vi "Dashboard Main.vi"() -> ()   [LabVIEW 2019]
uses:
  <vilib>/Utility/miscctls.llb/LVRowAndColumnTypeDef.ctl
  <vilib>/event_ctls.llb/eventvkey.ctl
  <vilib>/Rock Robotics/Network Tables/NT Read Numeric Array.vi
  <vilib>/Rock Robotics/Network Tables/NT Write Numeric Array.vi
  <vilib>/Rock Robotics/Network Tables/NT Read Boolean.vi
  <vilib>/Rock Robotics/WPI/Dashboard/WPI_DashboardLogging Global.vi
panel:
  in  "Camera Settings Right":T1={"Frame Rate"=30, "Compression"=30, "Size"=1, "DB Camera Config"=FALSE} {"Frame Rate" scale=1.0..30.0; "Compression" scale=100.0..-1.0; "Size" items=["640x480", "320x240", "160x120"]}
  in  "Camera Name Right":string(combo)="No Camera Selection"
  out "Camera Perf":string
  in  "Camera Settings":T1={"Frame Rate"=30, "Compression"=30, "Size"=1, "DB Camera Config"=FALSE} {"Frame Rate" scale=1.0..30.0; "Compression" scale=100.0..-1.0; "Size" items=["640x480", "320x240", "160x120"]}
  in  "TCP":refnum<k5>
  in  "Rec Mode":enum32{"Stop", "Record", "Playback"}(radio)
  out "Image Message":string="Timeout in Camera Communications"
  in  "Dashboard Tab":T2(tab)
  in  "Position":enum16{"", "1", "2", "3"}(ring)
  in  "Auto Route":string(combo)
  out "VisionAligned":bool
  out "NT Connection":bool
  out "Mode":T3(ring)=enum."Auto Disabled"
  out "Right Camera Perf":cluster{"Bandwidth (Mbps)":dbl, "FPS":dbl}
  in  "Write Swerve Offsets":bool
  out "Camera Image Right":T4(plugin-control)
  in  "DB/String 9":string
  in  "DB/String 8":string
  in  "DB/String 7":string
  in  "DB/String 6":string
  in  "DB/String 5":string
  in  "DB/String 4":string
  in  "DB/String 3":string
  in  "DB/String 2":string
  in  "DB/String 1":string
  in  "DB/String 0":string
  in  "DB/Slider 0":dbl(slide) scale=0.0..5.0
  in  "DB/Slider 1":dbl(slide) scale=0.0..5.0
  in  "DB/Slider 2":dbl(slide) scale=0.0..5.0
  in  "DB/Slider 3":dbl(slide) scale=0.0..5.0
  out "DB/LED 3":bool
  out "DB/LED 2":bool
  out "DB/LED 1":bool
  out "DB/LED 0":bool
  in  "DB/Button 3":bool
  in  "DB/Button 2":bool
  in  "DB/Button 1":bool
  in  "DB/Button 0":bool caption="New Name"
  in  "Test Slider":dbl(slide) scale=0.0..100.0 scale format="%#_3g"
  in  "On/Off":bool caption="Solenoid"
  in  "Test Name":u16(ring) items=["Select the test to run..."]
  in  "Test Tree":string(tree)
  in  "Motor":cluster{"Value":dbl, "Enable":bool} {"Value" scale=-1.0..1.0 scale format="%#_3g"}
  out "Progress":T5 {"Test Progress" scale=0.0..100.0}
  in  "Rev/Fwd":cluster{"Forward":bool, "Reverse":bool}
  in  "Test Ring":u16(ring) items=["Monochrome", "Color"]
  out "Cmd Status":string
  in  "Execute Command":bool
  in  "Command Params":string[][](table)
  in  "Command Selection":i32(listbox)
  in  "CheckList":i32(listbox)
  out "Tree":string(tree)
  out "Camera Image":T4(plugin-control)
  out "Background":bool
  in  "Camera Name":string(combo)="No Camera Selection"
  # "HW"
  # "HW"
  # "General"
  # "Autonomous"
  # "This tab is a great place for autonomous settings and robot-specific values.\nPlace controls and indicators inside this tab and match name to\nDashboard Variables on robot. You can also delete this comment."
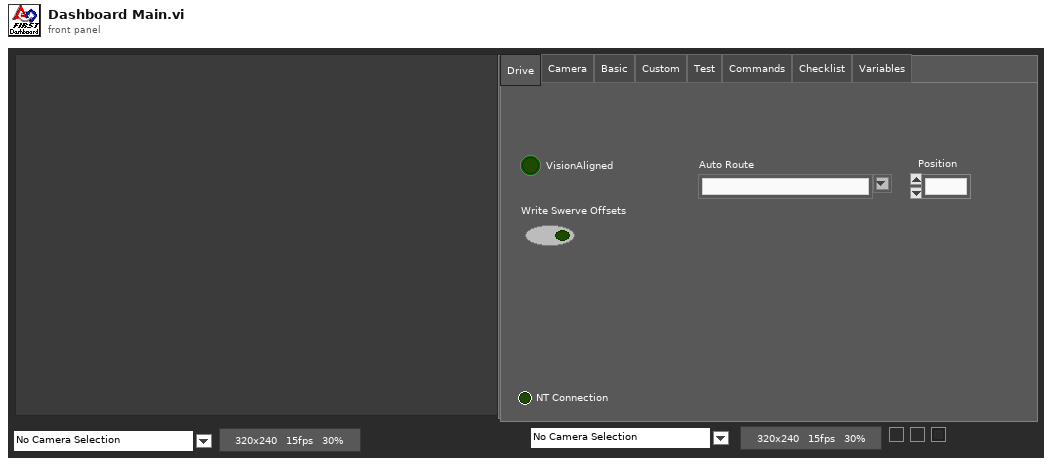
[diagram p1: front panel]
types:
  T1 = cluster{"Frame Rate":i32, "Compression":i32, "Size":u16, "DB Camera Config":bool}
  T2 = enum32{"Drive", "Camera", "Basic", "Custom", "Test", "Commands", "Checklist", "Variables"}
  T3 = enum8{"Tele-Op Disabled", "Tele-Op Enabled", "Auto Disabled", "Auto Enabled", "Test Disabled", "Test Enabled", "Disconnected", "No Code", "E-Stop"}
  T4 = typedef "IMAQ Image.ctl" = refnum<image>
  T5 = cluster{"Test Progress":u8, "Test Progress Text":string}
  T6 = cluster{"Save Path":path, "Interval (s)":dbl, "Keep":i32}
  T7 = typedef "Image Type" = u32
  T8 = cluster{"IDs":cluster{"RPC field ID":u16, "Unique ID":u16}, "String":string}
  T9 = cluster{"Camera Image":refnum<vi>, "Dashboard Tab":refnum<vi>, "Background":refnum<vi>, "Rec Mode":refnum<vi>, "Test Slider":refnum<vi>, "On/Off ":refnum<vi>, "Test Ring":refnum<vi>, "Rev/Fwd":refnum<vi>, "Test Name":refnum<vi>, "Motor":refnum<vi>, "Progress":refnum<vi>, "CheckList":refnum<vi>, "Tree":refnum<vi>, "Test Tree":refnum<vi>, "Command Params":refnum<vi>, "Command Selection":refnum<vi>, "Execute Command":refnum<vi>, "Cmd Status":refnum<vi>, "Camera Settings":refnum<vi>, "Camera Name":refnum<vi>, "Camera Perf":refnum<vi>, "Camera Settings Right":refnum<vi>, "Camera Name Right":refnum<vi>, "Camera Image Right":refnum<vi>}
  T10 = cluster{"Global Rectangle":i32[], "Contours":cluster{"Contour Type":u32, "ROI Type":u32, "Points":i32[]}[]}
  T11 = cluster{"Camera Name":string, string, "Saved DB Images Info":cluster{"Save Path":path, "Interval (s)":dbl, "Keep":i32}}
  T12 = cluster{"Camera Name Right":string, string, "Saved DB Images Info":cluster{"Save Path":path, "Interval (s)":dbl, "Keep":i32}}
  T13 = cluster{"Operation":enum16{"Update", "Clear"}, "Color Box":u32}[]
  T14 = typedef "eventvkey.ctl" = enum16{"ASCII", "Enter", "Return", "Shift", "Ctrl", "Alt", "Cmd", "Opt", "Caps", "NumLock", "Clear", "Break", "Up", "Down", "Left", "Right", "Insert", "Delete", "Home", "End", "PageUp", "PageDown", "Escape", "Help", "Pause", "ScrollLock", "F1", "F2", "F3", "F4", "F5", "F6", "F7", "F8", "F9", "F10", "F11", "F12", "F13", "F14", "F15", "F16", "F17", "F18", "F19", "F20", "F21", "F22", "F23", "F24", "Play", "VolumeUp", "VolumeDown", "Mute", "Two Byte Char"}
  T15 = cluster{"Image Size":bool, "Image Type":bool, "Pixel Value":bool, "ROI Information":bool, "Zoom Factor":bool}
  T16 = cluster{"Operation":enum16{"Update", "Clear"}, "Color Box":u32}
  T17 = typedef "LVRowAndColumnTypeDef.ctl" = cluster{"Row":i32, "Column":i32}
  T18 = cluster{"Shift":bool, "Ctrl":bool, "Alt":bool, "Cmd":bool, "Opt":bool}
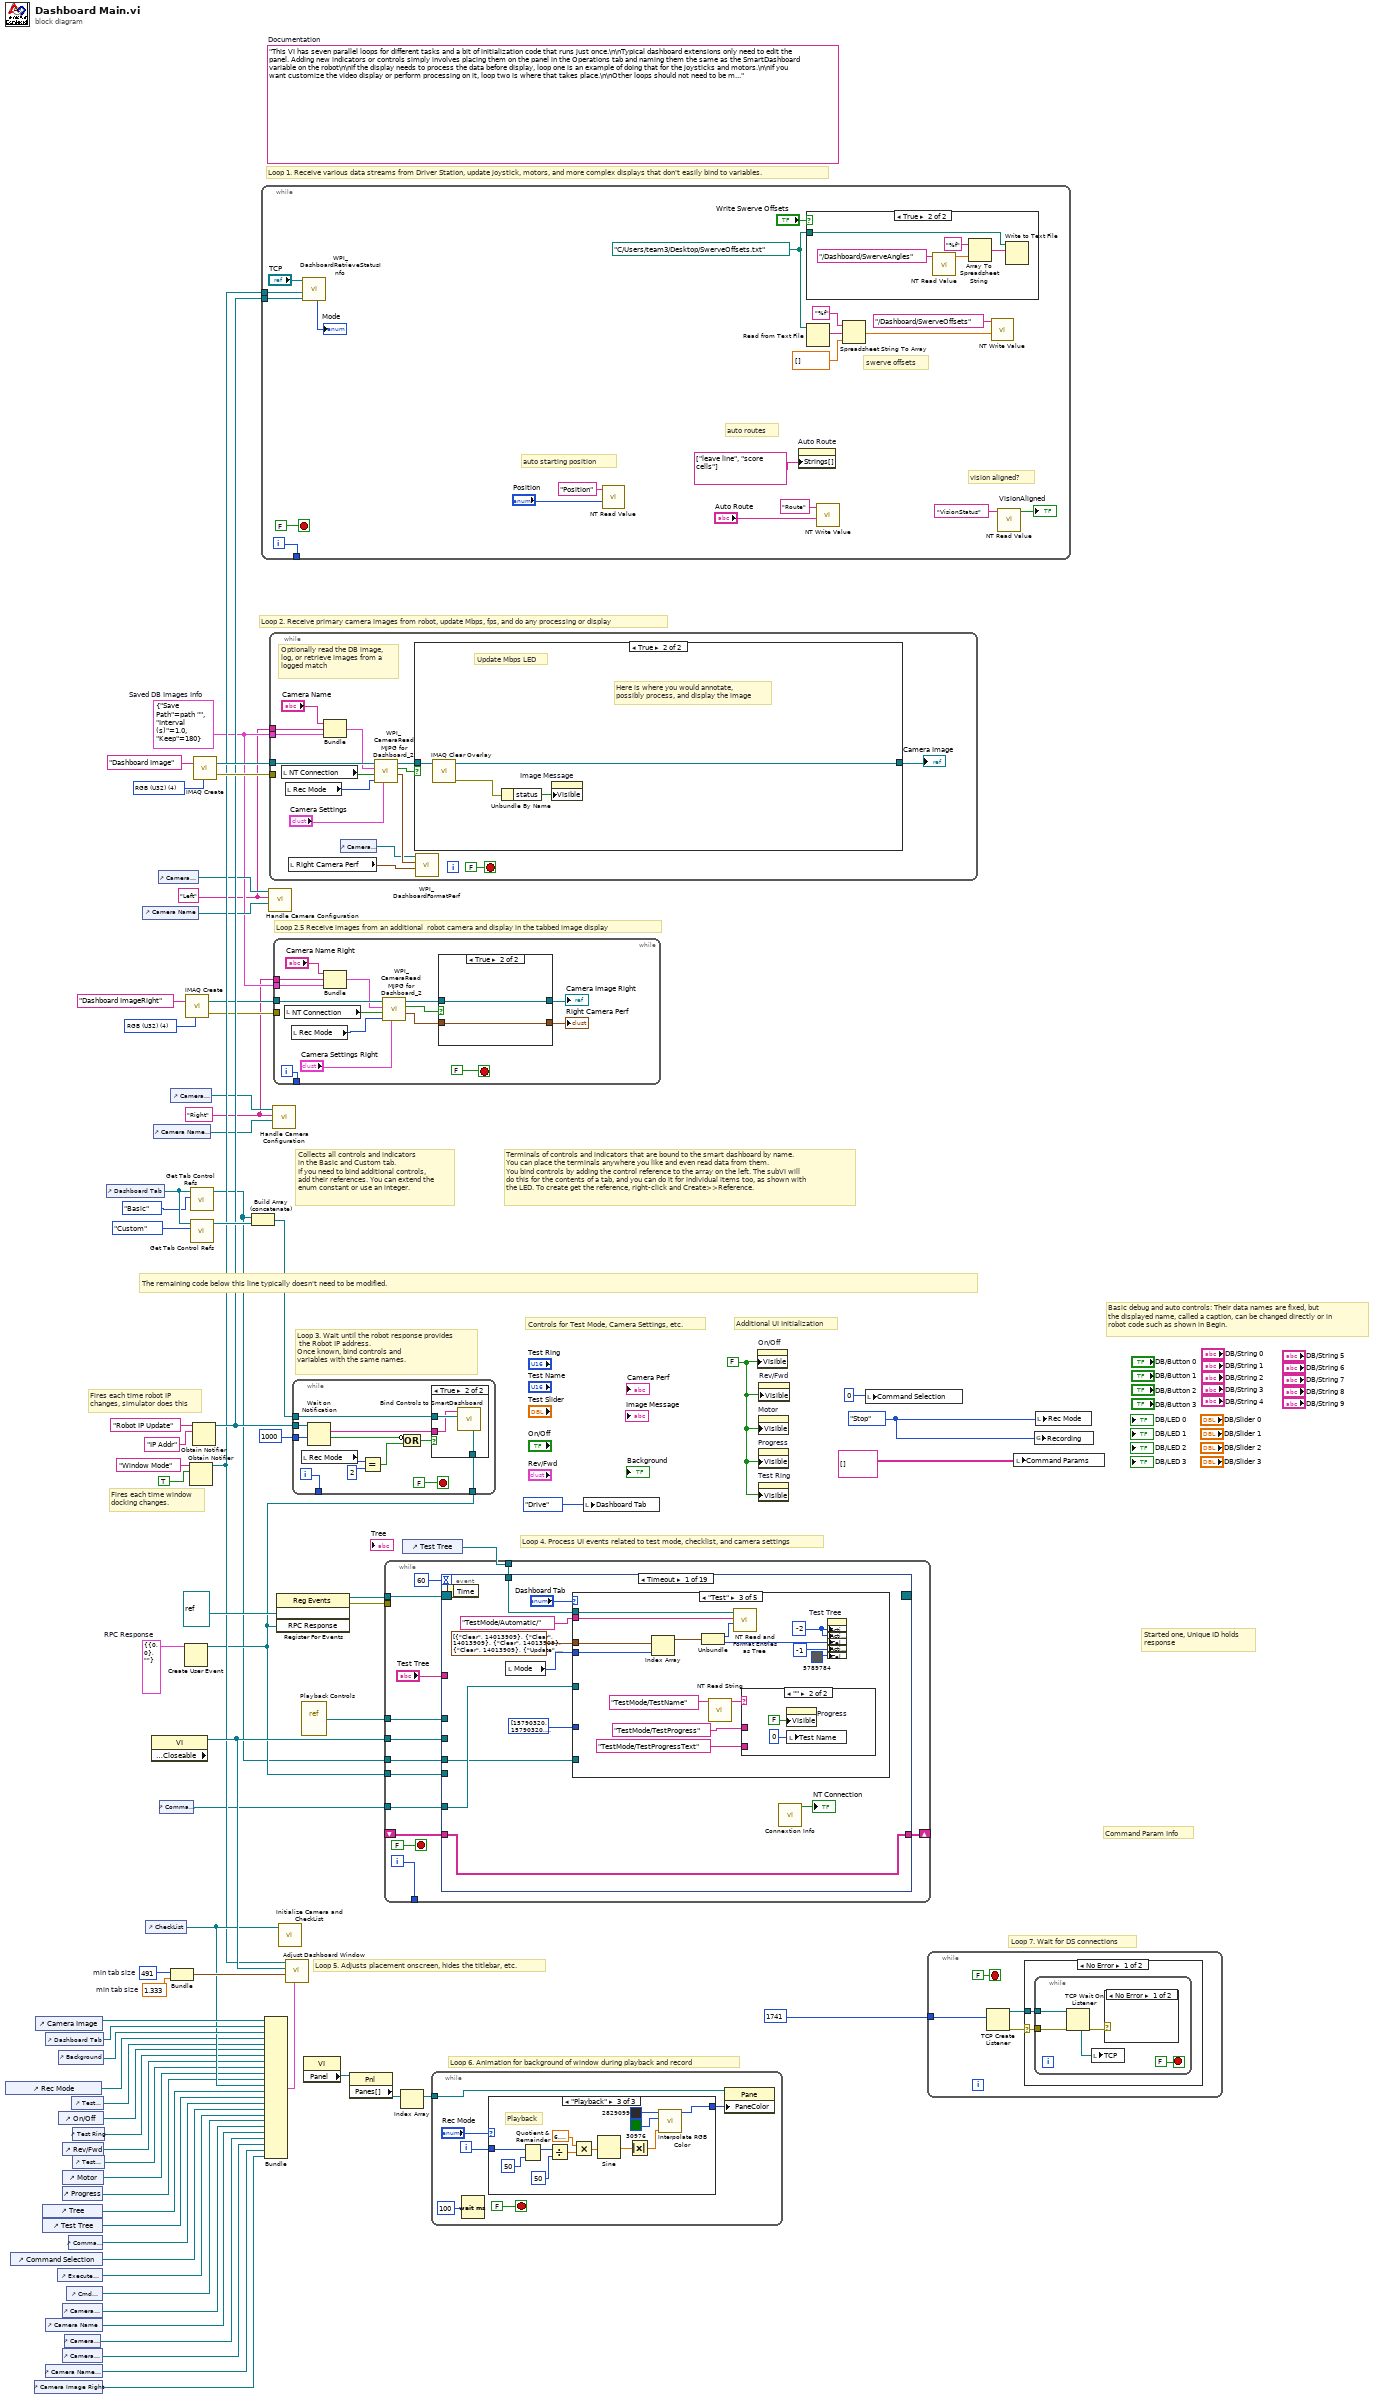
[diagram p0: block diagram]
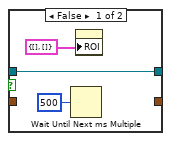
[diagram p2: hidden frame]
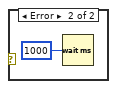
[diagram p3: hidden frame]
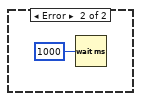
[diagram p4: hidden frame]
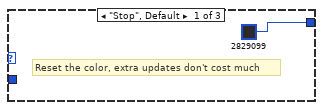
[diagram p6: hidden frame]
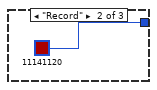
[diagram p7: hidden frame]
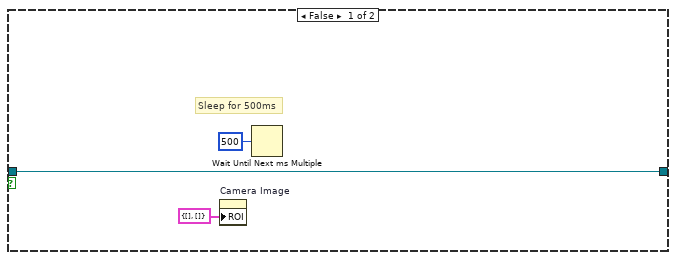
[diagram p9: hidden frame]
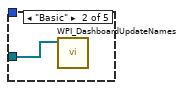
[diagram p11: hidden frame]
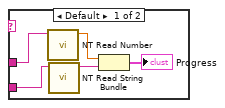
[diagram p12: hidden frame]
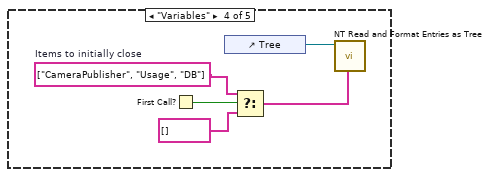
[diagram p13: hidden frame]
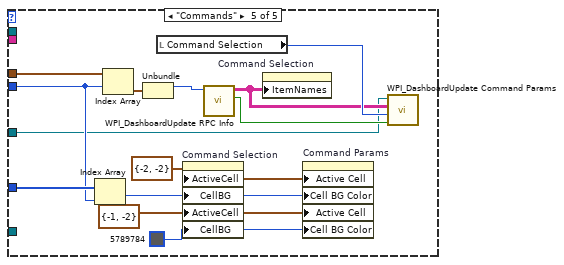
[diagram p14: hidden frame]
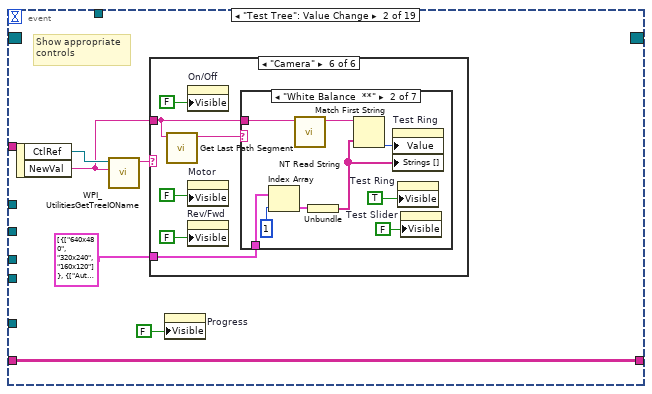
[diagram p15: hidden frame]
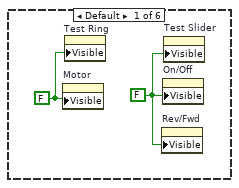
[diagram p16: hidden frame]
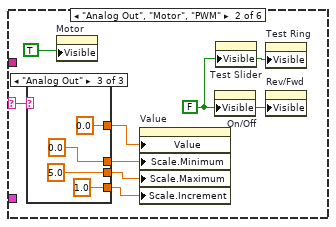
[diagram p17: hidden frame]
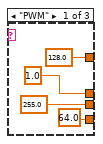
[diagram p18: hidden frame]
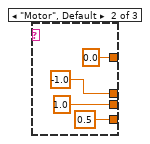
[diagram p19: hidden frame]
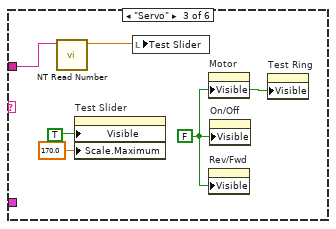
[diagram p20: hidden frame]
diagram:
  w3 = T6 {"Save Path"=path "", "Interval (s)"=1.0, "Keep"=180}  # Saved DB Images Info
  w2 = "Right"
  w1 = "Left"
  w13 = T7 4 items=["Grayscale (U8)", "Grayscale (I16)", "Grayscale (SGL)", "Complex (CSG)", "RGB (U32)", "HSL (U32)", "RGB (U64)"] ("Image Type")
  w27 = T8 {"IDs"={"RPC field ID"=0, "Unique ID"=0}, "String"=""}  # RPC Response
  w50 = 491  # min tab size
  w49 = 1.333  # min tab size
  w57 = enum32{"Stop", "Record", "Playback"}."Stop" ("Rec Mode")
  w34 = FALSE ("Visible")
  (unwired) "This VI has seven parallel loops for different tasks and a bit of initialization code that runs just once.\n\nTypical dashboard extensions only need to edit the panel. Adding new indicators or controls simply involves placing them on the panel in the Operations tab and naming them the same as the SmartDashboard variable on the robot\n\nIf the display needs to process the data before display, loop one is an example of doing that for the joysticks and motors.\n\nIf you want customize the video display or perform processing on it, loop two is where that takes place.\n\nOther loops should not need to be modified. They are pretty standard, and document the task they perform."  # Documentation
  w74 = T7 4 items=["Grayscale (U8)", "Grayscale (I16)", "Grayscale (SGL)", "Complex (CSG)", "RGB (U32)", "HSL (U32)", "RGB (U64)"] ("Image Type")
  # "Loop 2.5 Receive images from an additional  robot camera and display in the tabbed image display"
  # "Command Param Info"
  # "Started one, Unique ID holds\nresponse"
  # "Loop 7. Wait for DS connections"
  # "Basic debug and auto controls: Their data names are fixed, but\nthe displayed name, called a caption, can be changed directly or in\nrobot code such as shown in Begin."
  # "Controls for Test Mode, Camera Settings, etc."
  # "Additional UI Initialization"
  # "Loop 6. Animation for background of window during playback and record"
  # "Fires each time robot IP\nchanges, simulator does this"
  # "Fires each time window\ndocking changes."
  # "Collects all controls and indicators\nin the Basic and Custom tab.\nIf you need to bind additional controls,\nadd their references. You can extend the\nenum constant or use an integer."
  # "The remaining code below this line typically doesn't need to be modified."
  # "Loop 4. Process UI events related to test mode, checklist, and camera settings"
  # "Terminals of controls and indicators that are bound to the smart dashboard by name.\nYou can place the terminals anywhere you like and even read data from them.\nYou bind controls by adding the control reference to the array on the left. The subVI will\ndo this for the contents of a tab, and you can do it for individual items too, as shown with\nthe LED. To create get the reference, right-click and Create>>Reference."
  # "Loop 3. Wait until the robot response provides\n the Robot IP address.\nOnce known, bind controls and\nvariables with the same names."
  # "Loop 5. Adjusts placement onscreen, hides the titlebar, etc."
  # "Loop 1. Receive various data streams from Driver Station, update joystick, motors, and more complex displays that don't easily bind to variables."
  # "Loop 2. Receive primary camera images from robot, update Mbps, fps, and do any processing or display"
  n1 = control-ref of="Rec Mode"() -> (w40:refnum<vi>)
  n2 = control-ref of="Command Selection"() -> (w26:refnum<vi>)
  n3 = control-ref of="Camera Image Right"() -> (w6:refnum<vi>)
  n4 = control-ref of="Camera Image"() -> (w52:refnum<vi>)
  n5 = control-ref of="Tree"() -> (w44:refnum<vi>)
  n6 = control-ref of="Test Tree"() -> (w43:refnum<vi>)
  n7 = control-ref of="Dashboard Tab"() -> (w51:refnum<vi>)
  n8 = control-ref of="Camera Name"() -> (w17:refnum<vi>)
  n9 = control-ref of="Camera Name Right"() -> (w7:refnum<vi>)
  n10 = control-ref of="Execute Command"() -> (w28:refnum<vi>)
  n11 = control-ref of="Background"() -> (w47:refnum<vi>)
  n12 = control-ref of="On/Off"() -> (w38:refnum<vi>)
  n13 = control-ref of="Progress"() -> (w35:refnum<vi>)
  n14 = control-ref of="Camera Settings"() -> (w18:refnum<vi>)
  n15 = control-ref of="Camera Settings Right"() -> (w8:refnum<vi>)
  n16 = control-ref of="Rev/Fwd"() -> (w36:refnum<vi>)
  n17 = control-ref of="Motor"() -> (w41:refnum<vi>)
  n18 = control-ref of="Camera Perf"() -> (w16:refnum<vi>)
  n19 = control-ref of="Cmd Status"() -> (w22:refnum<vi>)
  n20 = control-ref of="Command Params"() -> (w29:refnum<vi>)
  n21 = control-ref of="Test Slider"() -> (w39:refnum<vi>)
  n22 = control-ref of="Test Ring"() -> (w37:refnum<vi>)
  n23 = control-ref of="Test Name"() -> (w42:refnum<vi>)
  n24 = control-ref of="Dashboard Tab"() -> (w55:refnum<vi>)
  n25 = control-ref of="Camera Name"() -> (w19:refnum<vi>)
  n26 = control-ref of="CheckList"() -> (w45:refnum<vi>)
  n27 = property class="VI" props=["Front Panel.Closeable"]() -> (reference out=w56:refnum<vi>)  [unwired: 2 in, 2 out]
  n28 = control-ref of="Camera Name Right"() -> (w9:refnum<vi>)
  n29 = control-ref of="Camera Settings"() -> (w20:refnum<vi>)
  n30 = control-ref of="Command Params"() -> (w21:refnum<vi>)
  n31 = control-ref of="Camera Settings Right"() -> (w10:refnum<vi>)
  n32 = Bundle("min tab size"=w50, "min tab size"=w49) -> (w48:cluster{"min tab size":i32, "min tab size":dbl})  [unwired: 1 in]
  n33 = Create User Event(user event datatype=w27) -> (user event=w23:refnum<user-event>)  [unwired: 1 in, 1 out]
  n34 = call "IMAQ Create"("Image Name"="Dashboard ImageRight", "Image Type"=w13) -> ("New Image"=w12:T4, "error out"=w11:errorcluster)  [unwired: 2 in, 1 out]
  n35 = Obtain Notifier(name (unnamed)="Window Mode", notification data type=TRUE) -> (notifier out=w32:refnum<notifier>)  [unwired: 2 in, 2 out]
  n36 = call <vilib>:"Get Tab Control Refs.vi"("Page Index"=T2."Basic" ("Dashboard Tab"), "TabControl in"=w55) -> ("ControlsOnPage"=w15:refnum<vi>[])  [unwired: 9 in]
  n37 = call <vilib>:"Get Tab Control Refs.vi"("Page Index"=T2."Custom" ("Dashboard Tab"), "TabControl in"=w55) -> ("ControlsOnPage"=w54:refnum<vi>[])  [unwired: 9 in]
  n38 = Obtain Notifier(name (unnamed)="Robot IP Update", notification data type="IP Addr" ("name (unnamed)")) -> (notifier out=w33:refnum<notifier>)  [unwired: 2 in, 2 out]
  n39 = call "IMAQ Create"("Image Name"="Dashboard Image", "Image Type"=w74) -> ("New Image"=w72:T4, "error out"=w71:errorcluster)  [unwired: 2 in, 1 out]
  n40 = Build Array (concatenate)(w15, w54) -> (w53:refnum<vi>[])
  n41 = while {
    tunnel: [w93] -> _
    tunnel: w33 -> [w92]
    tunnel: w32 -> [w89]
    i -> [w93]
    stop <- FALSE stop-if-true
    w82 = path "C:/Users/team3/Desktop/SwerveOffsets.txt" ("file (use dialog)")
    # "auto starting position"
    # "auto routes"
    # "vision aligned?"
    # "swerve offsets"
    n42 = call <vilib>:"WPI_DashboardRetrieveStatusInfo.vi"("Binding Refnum"=w92, "Window Mode Notifier"=w89, "TCP Cnx"="TCP") -> ("Robot Mode"=→"Mode":T3)  [unwired: 3 in, 5 out]
    n43 = call-poly <vilib>:"NT Read Value.vi"("Default Value"="Position", "Name"="Position") -> ()  [unwired: 8 in, 2 out]
    n44 = property on="Auto Route" class="CmbBox"("Strings[]"=string[] ["leave line", "score cells"] ("Strings []")) -> ()  [unwired: 2 in, 2 out]
    n45 = case shown="True" "Write Swerve Offsets" {
      tunnel: w82 -> [_ w98]
      frame False {
      }
      frame True {
        n46 = call-poly <vilib>:"NT Read Value.vi"("Name"="/Dashboard/SwerveAngles") -> ("Numeric Array"=w97:dbl[])  [unwired: 9 in, 1 out]
        n47 = Array To Spreadsheet String(array=w97, 3:"%f" ("format string")) -> (spreadsheet string=w96:string)  [unwired: 1 in]
        n48 = Write to Text File(file (use dialog)=w98, text=w96) -> ()  [unwired: 2 in, 3 out]
      }
    }
    n49 = Read from Text File(file (use dialog)=w82) -> (text=w86:string)  [unwired: 3 in, 3 out]
    n50 = call-poly <vilib>:"NT Write Value.vi"("String"="Auto Route", "Name"="Route") -> ()  [unwired: 9 in, 1 out]
    n51 = Spreadsheet String To Array(format string="%f", spreadsheet string=w86, array type (2D Dbl)=dbl[] []) -> (array=w85:dbl[])  [unwired: 1 in]
    n52 = call-poly <vilib>:"NT Write Value.vi"("Numeric Array"=w85, "Name"="/Dashboard/SwerveOffsets") -> ()  [unwired: 9 in, 1 out]
    n53 = call-poly <vilib>:"NT Read Value.vi"("Name"="VisionStatus") -> ("Boolean"=→"VisionAligned":bool)  [unwired: 9 in, 1 out]
  }
  n54 = Bundle("Camera Image"=w52, "Dashboard Tab"=w51, "Background"=w47, "Rec Mode"=w40, "Test Slider"=w39, "On/Off"=w38, "Test Ring"=w37, "Rev/Fwd"=w36, "Test Name"=w42, "Motor"=w41, "Progress"=w35, "CheckList"=w45, "Tree"=w44, "Test Tree"=w43, "Command Params"=w29, "Command Selection"=w26, "Execute Command"=w28, "Cmd Status"=w22, "Camera Settings"=w18, "Camera Name"=w17, "Camera Perf"=w16, "Camera Settings Right"=w8, "Camera Name Right"=w7, "Camera Image Right"=w6) -> (w46:T9)  [unwired: 1 in]
  n55 = call "Handle Camera Configuration.vi"("CameraNameRef"=w19, "Display Name"=w1, "ClusterRef"=w20) -> ()  [unwired: 9 in]
  n56 = while {
    tunnel: w72 -> [w113]
    tunnel: w71 -> [_]
    tunnel: w3 -> [w106]
    tunnel: w1 -> [w103]
    stop <- FALSE stop-if-true
    # "Optionally read the DB image,\nlog, or retrieve images from a\nlogged match"
    n57 = local read "NT Connection"() -> (w107:bool)
    n58 = local read "Rec Mode"() -> (w110:enum32{"Stop", "Record", "Playback"})
    n59 = local read "Right Camera Perf"() -> (w101:cluster{"Bandwidth (Mbps)":dbl, "FPS":dbl})
    n60 = Bundle("Camera Name"="Camera Name", w103, "Saved DB Images Info"=w106) -> (w105:T11)  [unwired: 1 in]
    n61 = control-ref of="Camera Perf"() -> (w100:refnum<vi>)
    n62 = call <vilib>:"WPI_CameraRead MJPG for Dashboard_2.vi"("Camera Settings"="Camera Settings", "Rec Mode"=w110, "NT Connection"=w107, "Capture Info"=w105, "Image in"=w113) -> ("perf info"=w102:cluster{"Bandwidth (Mbps)":dbl, "fps":dbl}, "Active"=w111:bool, "Image\\ out"=w112:T4)  [unwired: 4 in]
    n63 = case shown="True" w111 {
      tunnel: w112 -> [w116 w119]
      tunnel: [w116 w118] -> w108
      frame False {
        # "Sleep for 500ms"
        n64 = property on="Camera Image" class="ImageControl"("ROI"=T10 {"Global Rectangle"=[], "Contours"=[]}) -> ()  [unwired: 2 in, 2 out]
        n65 = Wait Until Next ms Multiple(millisecond multiple=u32 500) -> ()  [unwired: 1 out]
      }
      frame True {
        # "Here is where you would annotate,\npossibly process, and display the image"
        # "Update Mbps LED"
        n66 = call "IMAQ Clear Overlay"("Image"=w119) -> ("error out"=w120:errorcluster, "Image Out"=w118:T4)  [unwired: 2 in, 7 out]
        n67 = Unbundle By Name(w120) -> ("status"=w121:bool)
        n68 = property on="Image Message" class="Str"("Visible"=w121) -> ()  [unwired: 2 in, 2 out]
      }
    }
    "Camera Image" <- w108
    n69 = call <vilib>:"WPI_DashboardFormatPerf.vi"("Right Camera Perf"=w101, "Performance"=w102, "String in"=w100) -> ()  [unwired: 9 in]
  }
  n70 = call "Handle Camera Configuration.vi"("CameraNameRef"=w9, "Display Name"=w2, "ClusterRef"=w10) -> ()  [unwired: 9 in]
  n71 = while {
    tunnel: w12 -> [w136]
    tunnel: w11 -> [_]
    tunnel: [w131] -> _
    tunnel: w3 -> [w127]
    tunnel: w2 -> [w124]
    i -> [w131]
    stop <- FALSE stop-if-true
    n72 = local read "NT Connection"() -> (w128:bool)
    n73 = local read "Rec Mode"() -> (w135:enum32{"Stop", "Record", "Playback"})
    n74 = Bundle("Camera Name Right"="Camera Name Right", w124, "Saved DB Images Info"=w127) -> (w126:T12)  [unwired: 1 in]
    n75 = call <vilib>:"WPI_CameraRead MJPG for Dashboard_2.vi"("Camera Settings"="Camera Settings Right", "Rec Mode"=w135, "NT Connection"=w128, "Capture Info"=w126, "Image in"=w136) -> ("perf info"=w122:cluster{"Bandwidth (Mbps)":dbl, "fps":dbl}, "Active"=w130:bool, "Image\\ out"=w133:T4)  [unwired: 4 in]
    n76 = case shown="True" w130 {
      tunnel: w133 -> [w138 w141]
      tunnel: [w138 w141] -> w129
      tunnel: [_ w140] -> w123
      tunnel: w122 -> [_ w140]
      frame False {
        n77 = Wait Until Next ms Multiple(millisecond multiple=u32 500) -> ()  [unwired: 1 out]
        n78 = property on="Camera Image Right" class="ImageControl"("ROI"=T10 {"Global Rectangle"=[], "Contours"=[]}) -> ()  [unwired: 2 in, 2 out]
      }
      frame True {
      }
    }
    "Camera Image Right" <- w129
    "Right Camera Perf" <- w123
  }
  n79 = register-events(refnum<vi> refnum, w23) -> (reference out=w61:refnum<event-registration>, error out=w60:errorcluster)  [unwired: 2 in]
  n80 = call "Initialize Camera and CheckList.vi"("ListBox in"=w45) -> ()  [unwired: 11 in]
  n81 = call "Adjust Dashboard Window.vi"("Sizing Refnums"=w46, "Size Constraints"=w48, "VI"=w56, "WIn Mode"=w32) -> ()  [unwired: 8 in]
  n82 = while {
    tunnel: w53 -> [w153]
    tunnel: w33 -> [w151]
    tunnel: [w149] -> _
    tunnel: u32 1000 ("milliseconds to wait") -> [w148]
    tunnel: w23 -> [w142]
    i -> [w149]
    stop <- FALSE stop-if-true
    n83 = local read "Rec Mode"() -> (w144:enum32{"Stop", "Record", "Playback"})
    n84 = Wait on Notification(notifier=w151, timeout in ms (-1)=w148) -> (notification=w150:string, timed out?=w146:bool)  [unwired: 2 in, 2 out]
    n85 = Equal?(x=w144, y=u16 2 ("Rec Mode")) -> (x = y?=w145:bool)
    n86 = Compound Arithmetic op=OR(invert w146, w145) -> (w147:bool)
    n87 = case shown="True" w147 {
      tunnel: w153 -> [_ w156]
      tunnel: w150 -> [_ w155]
      tunnel: w142 -> [_ w154]
      frame False {
      }
      frame True {
        n88 = call <vilib>:"Bind Controls to SmartDashboard.vi"("RPC ref"=w154, "Bound Control Refs"=w156, "Server IP Address"=w155) -> ()  [unwired: 9 in]
      }
    }
  }
  n89 = vi-ref "Playback Controls.vi"() -> (w62:refnum<vi>)
  n90 = property class="VI"() -> ("Panel"=w64:refnum<vi>)  [unwired: 2 in, 2 out]
  n91 = property class="Pnl"(reference=w64) -> ("Panes[]"=w65:refnum<vi>[])  [unwired: 1 in, 2 out]
  n92 = Index Array(array=w65) -> (element=w63:refnum<vi>)  [unwired: 1 in]
  n93 = control-ref of="Test Tree"() -> (w66:refnum<vi>)
  n94 = while {
    tunnel: [w166] -> _
    tunnel: w66 -> [w165]
    tunnel: w62 -> [w164]
    tunnel: w61 -> [w163]
    tunnel: w60 -> [_]
    tunnel: w56 -> [w162]
    tunnel: w23 -> [w161]
    tunnel: w21 -> [w160]
    shift-right: [w159] -> _
    shift-left: _ -> [w158]
    tunnel: w15 -> [w157]
    i -> [w166]
    stop <- FALSE stop-if-true
    n95 = event shown="[0] Timeout" {
      selector: w163 -> [_ _ _ _ _ _ _ _ _ _ _ _ _ _ _ _ _ _ _]
      dyn-events: [_ _ _ _ _ _ _ _ _ _ _ _ _ _ w420 _ _ _ _] -> _
      timeout: u32 60 ("milliseconds to wait") -> [_ _ _ _ _ _ _ _ _ _ _ _ _ _ _ _ _ _ _]
      tunnel: w165 -> [w178 _ _ _ _ _ _ _ _ _ _ _ _ _ _ _ _ _ _]
      tunnel: "Test Tree" -> [_ _ _ _ _ _ _ _ _ w387 w395 w397 w401 w409 _ _ _ _ _]
      tunnel: w164 -> [_ _ _ _ _ _ _ _ _ _ _ _ _ _ w422 _ w440 _ _]
      tunnel: w162 -> [_ _ _ _ _ _ _ _ _ _ _ _ _ _ w418 _ _ _ _]
      tunnel: w161 -> [_ _ _ _ _ _ _ _ _ _ _ _ _ _ w416 _ _ _ _]
      tunnel: w160 -> [w173 _ _ _ w338 _ _ _ _ _ _ _ _ _ _ _ _ _ _]
      tunnel: [w172 w221 w323 w328 w336 w345 w355 w362 w374 w386 w393 w396 w400 w408 w415 w435 w437 w441 w454] -> w159
      tunnel: w158 -> [w172 w221 w323 w328 w336 _ _ w362 w374 w386 w393 w396 w400 w408 w415 w435 w437 w441 w454]
      tunnel: w157 -> [w170 _ _ _ _ _ _ _ _ _ _ _ _ _ _ _ _ _ _]
      event Timeout {
        n96 = event-data() -> ()  [unwired: 1 in, 1 out]
        n97 = local read "Mode"() -> (w175:T3)
        n98 = case shown="\"Test\"" "Dashboard Tab" {
          tunnel: w178 -> [_ _ w194 _ _]
          tunnel: "TestMode/Automatic/" ("Name Pattern") -> [_ _ w193 _ _]
          tunnel: T13 [{"Operation"=enum."Clear", "Color Box"=14013909}, {"Operation"=enum."Clear", "Color Box"=14013909}, {"Operation"=enum."Clear", "Color Box"=14013909}, {"Operation"=enum."Clear", "Color Box"=14013909}, {"Operation"=enum."Update", "Color Box"=14013909}, {"Operation"=enum."Update", "Color Box"=16777215}, {"Operation"=enum."Clear", "Color Box"=14013909}, {"Operation"=enum."Clear", "Color Box"=14013909}, {"Operation"=enum."Clear", "Color Box"=14013909}] -> [_ _ w186 _ w214]
          tunnel: w175 -> [_ _ w185 _ w213]
          tunnel: u32[] [15790320, 15790320, 15790320, 15790320, 16777215, 16777215, 15790320, 15790320, 15790320] -> [_ _ _ _ w219]
          tunnel: w173 -> [_ _ _ _ w207]
          tunnel: w170 -> [_ w180 _ _ _]
          frame "Custom", Default {
          }
          frame "Basic" {
            n99 = call <vilib>:"WPI_DashboardUpdateNames.vi"("Controls on Tab"=w180) -> ()  [unwired: 11 in]
          }
          frame "Test" {
            w192 = -2 ("Active Item:Row Number")
            n100 = Index Array(array=w186, index=w185) -> (element=w187:T16)
            n101 = Unbundle(w187) -> ("Operation"=w188:enum16{"Update", "Clear"}, "Color Box"=w189:u32)
            n102 = call <vilib>:"NT Read String.vi"("Name"="TestMode/TestName") -> ("String"=w183:string)  [unwired: 9 in, 1 out]
            n103 = call <vilib>:"NT Read and Format Entries as Tree.vi"("Operation"=w188, "Name Pattern"=w193, "Tree Refnum"=w194) -> ()  [unwired: 7 in, 2 out]
            n104 = case shown="\"\"" w183 {
              tunnel: "TestMode/TestProgress" ("Name") -> [w196 _]
              tunnel: "TestMode/TestProgressText" ("Name") -> [w195 _]
              frame Default {
                n105 = call <vilib>:"NT Read Number.vi"("Name"=w196) -> ("Numeric"=w197:dbl)  [unwired: 9 in, 1 out]
                n106 = call <vilib>:"NT Read String.vi"("Name"=w195) -> ("String"=w198:string)  [unwired: 9 in, 1 out]
                n107 = Bundle("Numeric"=w197, "String"=w198) -> (→"Progress":cluster{"Numeric":dbl, "String":string})  [unwired: 1 in]
              }
              frame "" {
                n108 = property on="Progress" class="Clust (strict)"("Visible"=FALSE) -> ()  [unwired: 2 in, 2 out]
                n109 = local write "Test Name"(u16 0) -> ()
              }
            }
            n110 = property on="Test Tree" class="Tree (strict)"("Active Item Row Number"=w192, "ActiveColNum"=w192, "CellBG"=w189, "Active Item Row Number"=-1 ("Active Item:Row Number"), "CellBG"=u32 5789784 ("Color Box")) -> ()  [unwired: 2 in, 2 out]
          }
          frame "Variables" {
            w204 = string[] ["CameraPublisher", "Usage", "DB"]  # Items to initially close
            n111 = First Call?() -> (First Call?: T/F=w205:bool)
            n112 = control-ref of="Tree"() -> (w206:refnum<vi>)
            n113 = Select(t=w204, s=w205, f=string[] []) -> (s? t:f=w202:string[])
            n114 = call <vilib>:"NT Read and Format Entries as Tree.vi"("Tags to  Close"=w202, "Tree Refnum"=w206) -> ()  [unwired: 8 in, 2 out]
          }
          frame "Commands" {
            w215 = u32 5789784 ("Color Box")
            w216 = T17 {"Row"=-1, "Column"=-2} ("Active Cell:Active Cell")
            w218 = T17 {"Row"=-2, "Column"=-2} ("Active Cell:Active Cell")
            n115 = Index Array(array=w219, index=w213) -> (element=w217:u32)
            n116 = Index Array(array=w214, index=w213) -> (element=w212:T16)
            n117 = Unbundle(w212) -> ("Operation"=w211:enum16{"Update", "Clear"})  [unwired: 1 out]
            n118 = local read "Command Selection"() -> (w210:i32)
            n119 = property on="Command Selection" class="MCListbox (strict)"("ActiveCell"=w218, "CellBG"=w217, "ActiveCell"=w216, "CellBG"=w215) -> ()  [unwired: 2 in, 2 out]
            n120 = call <vilib>:"WPI_DashboardUpdate RPC Info.vi"("Operation"=w211) -> ("update"=w209:bool, "commands"=w208:string[][])  [unwired: 9 in]
            n121 = property on="Command Selection" class="MCListbox (strict)"("ItemNames"=w208) -> ()  [unwired: 2 in, 2 out]
            n122 = property on="Command Params" class="Tbl (strict)"("Active Cell"=w218, "Cell BG Color"=w217, "Active Cell"=w216, "Cell BG Color"=w215) -> ()  [unwired: 2 in, 2 out]
            n123 = call <vilib>:"WPI_DashboardUpdate Command Params.vi"("Update"=w209, "NewVal"=w210, "Commands"=w208, "Param Tbl"=w207) -> ()  [unwired: 7 in, 1 out]
          }
        }
        n124 = call <vilib>:"Connextion Info.vi"() -> ("Connected"=→"NT Connection":bool)  [unwired: 10 in, 1 out]
      }
      event "Test Tree": Value Change {
        # "Show appropriate\ncontrols"
        n125 = event-data() -> ("CtlRef"=w224:refnum<vi>, "NewVal"=w222:string)  [unwired: 1 in]
        n126 = call <vilib>:"WPI_UtilitiesGetTreeIOName.vi"("NewVal"=w222, "TreeControl in"=w224) -> ("I/O Name"=w225:string)  [unwired: 9 in]
        n127 = case shown="\"Camera\"" w225 {
          selector: w225 -> [_ w232 _ w254 w263 _]
          tunnel: w222 -> [_ _ w251 w253 _ w270]
          tunnel: cluster{string[]}[] [{["640x480", "320x240", "160x120"]}, {["Auto", "Fixed indoor", "Fixed outdoor 1", "Fixed outdoor 2", "Fixed fluorescent 1", "Fixed fluorescent 2", "Hold current"]}, {["Auto", "Flicker-free 50 Hz", "Flicker-free 60 Hz", "Hold current"]}, {["None", "Prioritize frame rate", "Prioritize image quality"]}, {["Monochrome", "Color"]}] -> [_ _ _ _ _ w269]
          frame Default {
            w227 = FALSE ("Visible")
            w226 = FALSE ("Visible")
            n128 = property on="Motor" class="Clust (strict)"("Visible"=w226) -> ()  [unwired: 2 in, 2 out]
            n129 = property on="Test Ring" class="Ring (strict)"("Visible"=w226) -> ()  [unwired: 2 in, 2 out]
            n130 = property on="Rev/Fwd" class="Clust (strict)"("Visible"=w227) -> ()  [unwired: 2 in, 2 out]
            n131 = property on="On/Off" class="Bool (strict)"("Visible"=w227) -> ()  [unwired: 2 in, 2 out]
            n132 = property on="Test Slider" class="Slide (strict)"("Visible"=w227) -> ()  [unwired: 2 in, 2 out]
          }
          frame "Analog Out", "Motor", "PWM" {
            w233 = FALSE ("Visible")
            n133 = case shown="\"Analog Out\"" w232 {
              tunnel: [1.0 ("Value") -1.0 ("Value") 0.0 ("Value")] -> w231
              tunnel: [255.0 ("Value") 1.0 ("Value") 5.0 ("Value")] -> w230
              tunnel: [128.0 ("Value") 0.0 ("Value") 0.0 ("Value")] -> w229
              tunnel: [64.0 ("Value") 0.5 ("Value") 1.0 ("Value")] -> w228
              frame "PWM" {
              }
              frame "Motor", Default {
              }
              frame "Analog Out" {
              }
            }
            n134 = property on="Motor" class="Clust (strict)"("Visible"=TRUE) -> ()  [unwired: 2 in, 2 out]
            n135 = property on="Value" class="Slide (strict)"("Value"=w229, "Scale.Minimum"=w231, "Scale.Maximum"=w230, "Scale.Increment"=w228) -> ()  [unwired: 2 in, 2 out]
            n136 = property on="On/Off" class="Bool (strict)"("Visible"=w233) -> ()  [unwired: 2 in, 2 out]
            n137 = property on="Test Slider" class="Slide (strict)"("Visible"=w233) -> ()  [unwired: 2 in, 2 out]
            n138 = property on="Test Ring" class="Ring (strict)"("Visible"=w233) -> ()  [unwired: 2 in, 2 out]
            n139 = property on="Rev/Fwd" class="Clust (strict)"("Visible"=w233) -> ()  [unwired: 2 in, 2 out]
          }
          frame "Servo" {
            w249 = FALSE ("Visible")
            n140 = call <vilib>:"NT Read Number.vi"("Name"=w251) -> ("Numeric"=w250:dbl)  [unwired: 9 in, 1 out]
            n141 = property on="Test Slider" class="Slide (strict)"("Visible"=TRUE, "Scale.Maximum"=170.0 ("Scale.Range:Maximum")) -> ()  [unwired: 2 in, 2 out]
            n142 = local write "Test Slider"(w250) -> ()
            n143 = property on="Motor" class="Clust (strict)"("Visible"=w249) -> ()  [unwired: 2 in, 2 out]
            n144 = property on="Rev/Fwd" class="Clust (strict)"("Visible"=w249) -> ()  [unwired: 2 in, 2 out]
            n145 = property on="On/Off" class="Bool (strict)"("Visible"=w249) -> ()  [unwired: 2 in, 2 out]
            n146 = property on="Test Ring" class="Ring (strict)"("Visible"=w249) -> ()  [unwired: 2 in, 2 out]
          }
          frame "Relay", "Solenoid" {
            w252 = FALSE ("Visible")
            n147 = property on="Motor" class="Clust (strict)"("Visible"=w252) -> ()  [unwired: 2 in, 2 out]
            n148 = property on="Test Slider" class="Slide (strict)"("Visible"=w252) -> ()  [unwired: 2 in, 2 out]
            n149 = Search and Replace String(input string=w253, search string="/Value  **", replace string="/Direction") -> (result string=w259:string)  [unwired: 5 in, 3 out]
            n150 = property on="Test Ring" class="Ring (strict)"("Visible"=w252) -> ()  [unwired: 2 in, 2 out]
            n151 = call <vilib>:"NT Read String.vi"("Name"=w259) -> ("String"=w257:string)  [unwired: 9 in, 1 out]
            n152 = Equal?(x="Both directions", y=w257) -> (x = y?=w255:bool)
            n153 = Not(x=w255) -> (.not. x?=w256:bool)
            n154 = property on="Rev/Fwd" class="Clust (strict)"("Visible"=w255) -> ()  [unwired: 2 in, 2 out]
            n155 = property on="On/Off" class="Bool (strict)"("Visible"=w256, "Caption.Text"=w254) -> ()  [unwired: 2 in, 2 out]
          }
          frame "Compressor", "Digital Out" {
            w262 = FALSE ("Visible")
            # "Get direction and finish"
            n156 = property on="Motor" class="Clust (strict)"("Visible"=w262) -> ()  [unwired: 2 in, 2 out]
            n157 = property on="Test Slider" class="Slide (strict)"("Visible"=w262) -> ()  [unwired: 2 in, 2 out]
            n158 = property on="Test Ring" class="Ring (strict)"("Visible"=w262) -> ()  [unwired: 2 in, 2 out]
            n159 = property on="On/Off" class="Bool (strict)"("Visible"=TRUE, "Caption.Text"=w263) -> ()  [unwired: 2 in, 2 out]
            n160 = property on="Rev/Fwd" class="Clust (strict)"("Visible"=FALSE) -> ()  [unwired: 2 in, 2 out]
          }
          frame "Camera" {
            n161 = call <vilib>:"Get Last Path Segment.vi"("String in"=w270) -> ("String out"=w271:string)  [unwired: 10 in]
            n162 = property on="On/Off" class="Bool (strict)"("Visible"=FALSE) -> ()  [unwired: 2 in, 2 out]
            n163 = property on="Motor" class="Clust (strict)"("Visible"=FALSE) -> ()  [unwired: 2 in, 2 out]
            n164 = property on="Rev/Fwd" class="Clust (strict)"("Visible"=FALSE) -> ()  [unwired: 2 in, 2 out]
            n165 = case shown="\"White Balance  **\"" w271 {
              tunnel: w270 -> [w277 w286 w295 w304 w313 _ w319]
              tunnel: w269 -> [w275 w283 w292 w301 w310 _ _]
              frame "Size  **" {
                n166 = Index Array(array=w275) -> (element=w274:cluster{string[]})  [unwired: 1 in]
                n167 = call <vilib>:"NT Read String.vi"("Name"=w277) -> ("String"=w276:string)  [unwired: 9 in, 1 out]
                n168 = Unbundle(w274) -> (w272:string[])
                n169 = Match First String(2:w272, 3:w276) -> (0:w273:i32)  [unwired: 1 out]
                n170 = property on="Test Ring" class="Ring (strict)"("Value"=w273, "Strings []"=w272) -> ()  [unwired: 2 in, 2 out]
                n171 = property on="Test Ring" class="Ring (strict)"("Visible"=TRUE) -> ()  [unwired: 2 in, 2 out]
                n172 = property on="Test Slider" class="Slide (strict)"("Visible"=FALSE) -> ()  [unwired: 2 in, 2 out]
              }
              frame "White Balance  **" {
                n173 = Index Array(array=w283, index=1) -> (element=w284:cluster{string[]})
                n174 = call <vilib>:"NT Read String.vi"("Name"=w286) -> ("String"=w285:string)  [unwired: 9 in, 1 out]
                n175 = Unbundle(w284) -> (w281:string[])
                n176 = Match First String(2:w281, 3:w285) -> (0:w280:i32)  [unwired: 1 out]
                n177 = property on="Test Ring" class="Ring (strict)"("Value"=w280, "Strings []"=w281) -> ()  [unwired: 2 in, 2 out]
                n178 = property on="Test Ring" class="Ring (strict)"("Visible"=TRUE) -> ()  [unwired: 2 in, 2 out]
                n179 = property on="Test Slider" class="Slide (strict)"("Visible"=FALSE) -> ()  [unwired: 2 in, 2 out]
              }
              frame "Exposure  **" {
                n180 = Index Array(array=w292, index=2) -> (element=w293:cluster{string[]})
                n181 = call <vilib>:"NT Read String.vi"("Name"=w295) -> ("String"=w294:string)  [unwired: 9 in, 1 out]
                n182 = Unbundle(w293) -> (w289:string[])
                n183 = Match First String(2:w289, 3:w294) -> (0:w290:i32)  [unwired: 1 out]
                n184 = property on="Test Ring" class="Ring (strict)"("Value"=w290, "Strings []"=w289) -> ()  [unwired: 2 in, 2 out]
                n185 = property on="Test Ring" class="Ring (strict)"("Visible"=TRUE) -> ()  [unwired: 2 in, 2 out]
                n186 = property on="Test Slider" class="Slide (strict)"("Visible"=FALSE) -> ()  [unwired: 2 in, 2 out]
              }
              frame "Exposure Priority  **" {
                n187 = Index Array(array=w301, index=3) -> (element=w302:cluster{string[]})
                n188 = call <vilib>:"NT Read String.vi"("Name"=w304) -> ("String"=w303:string)  [unwired: 9 in, 1 out]
                n189 = Unbundle(w302) -> (w298:string[])
                n190 = Match First String(2:w298, 3:w303) -> (0:w299:i32)  [unwired: 1 out]
                n191 = property on="Test Ring" class="Ring (strict)"("Value"=w299, "Strings []"=w298) -> ()  [unwired: 2 in, 2 out]
                n192 = property on="Test Ring" class="Ring (strict)"("Visible"=TRUE) -> ()  [unwired: 2 in, 2 out]
                n193 = property on="Test Slider" class="Slide (strict)"("Visible"=FALSE) -> ()  [unwired: 2 in, 2 out]
              }
              frame "Color Enable  **" {
                n194 = Index Array(array=w310, index=4) -> (element=w311:cluster{string[]})
                n195 = call <vilib>:"NT Read String.vi"("Name"=w313) -> ("String"=w312:string)  [unwired: 9 in, 1 out]
                n196 = Unbundle(w311) -> (w307:string[])
                n197 = Match First String(2:w307, 3:w312) -> (0:w308:i32)  [unwired: 1 out]
                n198 = property on="Test Ring" class="Ring (strict)"("Value"=w308, "Strings []"=w307) -> ()  [unwired: 2 in, 2 out]
                n199 = property on="Test Ring" class="Ring (strict)"("Visible"=TRUE) -> ()  [unwired: 2 in, 2 out]
                n200 = property on="Test Slider" class="Slide (strict)"("Visible"=FALSE) -> ()  [unwired: 2 in, 2 out]
              }
              frame Default {
                n201 = property on="Test Ring" class="Ring (strict)"("Visible"=FALSE) -> ()  [unwired: 2 in, 2 out]
                n202 = property on="Test Slider" class="Slide (strict)"("Visible"=FALSE) -> ()  [unwired: 2 in, 2 out]
              }
              frame "Brightness  **", "Color Level  **", "Compression  **", "FPS  **", "Sharpness  **" {
                n203 = call <vilib>:"NT Read Number.vi"("Name"=w319) -> ("Numeric"=w318:dbl)  [unwired: 9 in, 1 out]
                n204 = local write "Test Slider"(w318) -> ()
                n205 = property on="Test Slider" class="Slide (strict)"("Visible"=TRUE, "Scale.Maximum"=100.0 ("Scale.Range:Maximum")) -> ()  [unwired: 2 in, 2 out]
                n206 = property on="Test Ring" class="Ring (strict)"("Visible"=FALSE) -> ()  [unwired: 2 in, 2 out]
              }
            }
          }
        }
        n207 = property on="Progress" class="Clust (strict)"("Visible"=FALSE) -> ()  [unwired: 2 in, 2 out]
      }
      event "Test Name": Mouse Enter {
        # "Populate the ring with the list of tests"
        n208 = event-data() -> ()  [unwired: 1 in, 1 out]
        n209 = call <vilib>:"NT Read String Array.vi"("Name"="TestMode/TestList") -> ("String Array"=w327:string[])  [unwired: 9 in, 1 out]
        n210 = Build Array (concatenate)("Select the test to run...", w327) -> (w326:string[])
        n211 = property on="Test Name" class="Ring (strict)"("Strings []"=w326) -> ()  [unwired: 2 in, 2 out]
      }
      event "Test Name": Value Change {
        w329 = FALSE ("Visible")
        # "Tell the robot the test name to run"
        n212 = event-data() -> ("NewVal"=w333:u16)  [unwired: 1 in]
        n213 = property on="Test Name" class="Ring (strict)"() -> ("Strings []"=w334:string[])  [unwired: 2 in, 2 out]
        n214 = local write "Progress"(T5 {"Test Progress"=0, "Test Progress Text"=""} ("Progress")) -> ()
        n215 = Index Array(array=w334, index=w333) -> (element=w332:string)
        n216 = call <vilib>:"NT Write String.vi"("String"=w332, "Name"="TestMode/TestName") -> ()  [unwired: 9 in, 1 out]
        n217 = property on="Progress" class="Clust (strict)"("Visible"=TRUE) -> ()  [unwired: 2 in, 2 out]
        n218 = property on="Motor" class="Clust (strict)"("Visible"=w329) -> ()  [unwired: 2 in, 2 out]
        n219 = property on="Test Slider" class="Slide (strict)"("Visible"=w329) -> ()  [unwired: 2 in, 2 out]
        n220 = property on="On/Off" class="Bool (strict)"("Visible"=w329) -> ()  [unwired: 2 in, 2 out]
        n221 = property on="Rev/Fwd" class="Clust (strict)"("Visible"=w329) -> ()  [unwired: 2 in, 2 out]
        n222 = property on="Test Ring" class="Ring (strict)"("Visible"=w329) -> ()  [unwired: 2 in, 2 out]
      }
      event "Command Selection": Value Change {
        # "Get the params and show in table"
        n223 = event-data() -> ("NewVal"=w339:i32)  [unwired: 1 in]
        n224 = property on="Command Selection" class="MCListbox (strict)"() -> ("ItemNames"=w337:string[][])  [unwired: 2 in, 2 out]
        n225 = call <vilib>:"WPI_DashboardUpdate Command Params.vi"("NewVal"=w339, "Commands"=w337, "Param Tbl"=w338) -> ()  [unwired: 8 in, 1 out]
      }
      event "Execute Command": Value Change {
        # "Started one, Unique ID holds\nresponse"
        n226 = event-data() -> ()  [unwired: 1 in, 1 out]
        n227 = property on="Command Selection" class="MCListbox (strict)"() -> ("ItemNames"=w350:string[][])  [unwired: 2 in, 2 out]
        n228 = Index Array(array=w350, index (row)="Command Selection", index (col)=0) -> (element=w348:string)
        n229 = call <vilib>:"Invoke Commands.vi"("Command Params"="Command Params", "Function Name"=w348) -> ("Params"=w344:u8, "Started"=w343:bool)  [unwired: 7 in, 1 out]
        n230 = Array Subset(array="Command Params", length (row)=w344) -> (w345:string[][])  [unwired: 3 in]
        n231 = Select(t="Executing" ("Cmd Status"), s=w343, f="" ("Cmd Status")) -> (s? t:f=→"Cmd Status":string)
      }
      event "Command Selection": Double Click {
        n232 = event-data() -> ("Row"=w358:i32)  [unwired: 1 in]
        n233 = property on="Command Selection" class="MCListbox (strict)"() -> ("ItemNames"=w361:string[][])  [unwired: 2 in, 2 out]
        n234 = local read "Command Params"() -> (w357:string[][])
        n235 = Index Array(array=w361, index (row)=w358, index (col)=0) -> (element=w359:string)
        n236 = call <vilib>:"Invoke Commands.vi"("Command Params"=w357, "Function Name"=w359) -> ("Params"=w356:u8, "Started"=w351:bool)  [unwired: 7 in, 1 out]
        n237 = Array Subset(array=w357, length (row)=w356) -> (w355:string[][])  [unwired: 3 in]
        n238 = Select(t="Executing" ("Cmd Status"), s=w351, f="" ("Cmd Status")) -> (s? t:f=w352:string)
        n239 = local write "Cmd Status"(w352) -> ()
      }
      event "CheckList": Double Click {
        # "Shift clears all"
        # "Update symbols on the listbox"
        n240 = event-data() -> ("PlatMods.Shift"=w363:bool, "Row"=w365:i32)  [unwired: 1 in]
        n241 = case shown="True" w363 {
          tunnel: w365 -> [w369 _]
          tunnel: 1 -> [w368 _]
          frame False {
            n242 = property on="CheckList" class="LstBox (strict)"() -> ("Item Symbols"=w367:i32[])  [unwired: 2 in, 2 out]
            n243 = Replace Array Subset(array=w367, new element=w368, index=w369) -> (w366:i32[])
            n244 = property on="CheckList" class="LstBox (strict)"("Item Symbols"=w366) -> ()  [unwired: 2 in, 2 out]
          }
          frame True {
            w370 = 0 ("Top Row")
            n245 = property on="CheckList" class="LstBox (strict)"() -> ("Number of Rows"=w372:u32)  [unwired: 2 in, 2 out]
            n246 = Initialize Array(0, w372) -> (w371:i32[])
            n247 = property on="CheckList" class="LstBox (strict)"("Top Row"=w370, "Value"=w370, "Item Symbols"=w371) -> ()  [unwired: 2 in, 2 out]
          }
        }
      }
      event "CheckList": Key Down {
        # "Update symbols on the listbox\nLeft and right keys check and uncheck"
        n248 = event-data() -> ("VKey"=w376:T14)  [unwired: 1 in]
        n249 = case shown="\"Left\", \"Right\"" w376 {
          selector: w376 -> [w381 _]
          tunnel: eventvkey."Left" ("VKey") -> [w379 _]
          frame "Left", "Right" {
            n250 = Equal?(x=w379, y=w381) -> (x = y?=w380:bool)
            n251 = Select(t=0, s=w380, f=1) -> (s? t:f=w382:i32)
            n252 = property on="CheckList" class="LstBox (strict)"() -> ("Item Symbols"=w385:i32[])  [unwired: 2 in, 2 out]
            n253 = Replace Array Subset(array=w385, new element=w382, index="CheckList") -> (w384:i32[])
            n254 = property on="CheckList" class="LstBox (strict)"("Item Symbols"=w384) -> ()  [unwired: 2 in, 2 out]
          }
          frame Default {
          }
        }
      }
      event "Motor.Enable": Value Change {
        # "When the test mode otor enable helper is set, update that\ntree row item's value"
        n255 = event-data() -> ("NewVal"=w391:bool)  [unwired: 1 in]
        n256 = Unbundle("Motor") -> ("Value"=w390:dbl)  [unwired: 1 out]
        n257 = Select(t=w390, s=w391, f=0.0) -> (s? t:f=w388:dbl)
        n258 = call <vilib>:"NT Write Number.vi"("Numeric"=w388, "Name"=w387) -> ()  [unwired: 9 in, 1 out]
      }
      event "Test Slider": Value Change {
        # "When the test mode slider helper is set, update that\ntree row item's value"
        n259 = event-data() -> ("NewVal"=w394:dbl)  [unwired: 1 in]
        n260 = call <vilib>:"NT Write Number.vi"("Numeric"=w394, "Name"=w395) -> ()  [unwired: 9 in, 1 out]
      }
      event "On/Off": Value Change {
        # "When the test mode on/off helper value is set, update that\ntree row item's value"
        n261 = event-data() -> ("NewVal"=w399:bool)  [unwired: 1 in]
        n262 = Boolean To (0,1)(Boolean=w399) -> (0, 1=w398:i16)
        n263 = call <vilib>:"NT Write Number.vi"("Numeric"=w398, "Name"=w397) -> ()  [unwired: 9 in, 1 out]
      }
      event "Rev/Fwd": Value Change {
        # "When the test mode helper value for relays is set, update that\ntree row item's value"
        n264 = event-data() -> ("NewVal.Forward"=w407:bool, "NewVal.Reverse"=w406:bool)  [unwired: 1 in]
        n265 = Boolean To (0,1)(Boolean=w407) -> (0, 1=w403:i16)
        n266 = Boolean To (0,1)(Boolean=w406) -> (0, 1=w405:i16)
        n267 = Negate(x=w405) -> (-x=w404:i16)
        n268 = Add(x=w403, y=w404) -> (x+y=w402:i16)
        n269 = call <vilib>:"NT Write Number.vi"("Numeric"=w402, "Name"=w401) -> ()  [unwired: 9 in, 1 out]
      }
      event "Test Ring": Value Change {
        # "When a test mode helper value is selected from the ring,\nset the tree item's variable to the string value"
        n270 = event-data() -> ("NewVal"=w411:u16)  [unwired: 1 in]
        n271 = property on="Test Ring" class="Ring (strict)"() -> ("Strings []"=w412:string[])  [unwired: 2 in, 2 out]
        n272 = Index Array(array=w412, index=w411) -> (element=w410:string)
        n273 = call <vilib>:"NT Write String.vi"("String"=w410, "Name"=w409) -> ()  [unwired: 9 in, 1 out]
      }
      event "Rec Mode": Value Change {
        # "Update globals for recording mode and path to read log from.\nClear when logging and let NetworkTables set path for vision to\nuse."
        n274 = event-data() -> ("NewVal"=w423:enum32{"Stop", "Record", "Playback"})  [unwired: 1 in]
        n275 = global write "WPI_DashboardLogging Global.vi" "Logging Filename"(path "") -> ()
        n276 = global write "WPI_DashboardLogging Global.vi" "Recording"(w423) -> ()
        n277 = case shown="\"Playback\"" w423 {
          tunnel: w422 -> [_ w425 w434]
          tunnel: [_ _ w433] -> w420
          tunnel: [_ _ w432] -> _
          tunnel: w418 -> [_ _ w430]
          tunnel: cluster{i32, i32} {-250, 170} -> [_ _ w429]
          tunnel: [_ _ T15 {"Image Size"=TRUE, "Image Type"=TRUE, "Pixel Value"=TRUE, "ROI Information"=TRUE, "Zoom Factor"=FALSE} ("Image Information Shown:All Elements")] -> w413
          tunnel: [_ _ TRUE ("Zoom Factor")] -> w414
          tunnel: w416 -> [_ _ w426]
          frame Default {
          }
          frame "Stop", "Record" {
            # "Place Window too"
            n278 = invoke class="VI" method="FP.Close"(reference=w425) -> (reference out=w424:refnum<vi>)  [unwired: 2 in, 2 out]
            n279 = invoke class="VI" method="Abort VI"(reference=w424) -> ()  [unwired: 2 in, 3 out]
          }
          frame "Playback" {
            n280 = call "Open Playback Panel.vi"("Offset"=w429, "DB VI Ref"=w430, "Playback in"=w434) -> ("Playback out"=w431:refnum<vi>)  [unwired: 8 in]
            n281 = register-events(w431, w426) -> (reference out=w433:refnum<event-registration>, error out=w432:errorcluster)  [unwired: 2 in]
          }
        }
        n282 = property on="Camera Image Right" class="ImageControl"("Image Information Shown"=w413, "Image Information Visible"=w414) -> ()  [unwired: 2 in, 2 out]
        n283 = property on="Camera Image" class="ImageControl"("Image Information Shown"=w413, "Image Information Visible"=w414) -> ()  [unwired: 2 in, 2 out]
        n284 = call <vilib>:"WPI_DashboardNT Log FieldName Cache.vi"("Operation"=enum16{"Lookup/Add", "Index", "Clear"}."Clear") -> ()  [unwired: 8 in, 3 out]
      }
      event Panel Close {
        w436 = enum32{"Stop", "Record", "Playback"}."Stop" ("Rec Mode")
        # "Playback window has been closed, abort"
        n285 = event-data() -> ()  [unwired: 1 in, 4 out]
        n286 = local write "Rec Mode"(w436) -> ()
        n287 = global write "WPI_DashboardLogging Global.vi" "Recording"(w436) -> ()
      }
      event Panel Close {
        # "Abort playback window and ourself"
        n288 = event-data() -> ()  [unwired: 1 in, 4 out]
        n289 = invoke class="VI" method="FP.Close"(reference=w440) -> (reference out=w439:refnum<vi>)  [unwired: 2 in, 2 out]
        n290 = invoke class="VI" method="Abort VI"(reference=w439) -> (error out=w438:errorcluster)  [unwired: 2 in, 2 out]
        n291 = invoke class="VI" method="Abort VI"(error in=w438) -> ()  [unwired: 2 in, 3 out]
      }
      event User Event {
        n292 = event-data() -> ("IDs"=w447:cluster{"RPC field ID":u16, "Unique ID":u16}, "String"=w446:string)  [unwired: 1 in]
        n293 = Bundle("IDs"=w447, "String"=w446) -> (w445:T8)  [unwired: 1 in]
        n294 = call <vilib>:"Retrieve RPC Response.vi"("RPC Response"=w445) -> ("Output"=w443:string[][])  [unwired: 10 in]
        n295 = Build Array (concatenate)(w441, w443) -> (w442:string[][])
        n296 = local write "Command Params"(w442) -> ()
        n297 = local write "Cmd Status"("" ("Cmd Status")) -> ()
      }
      event "Tree": Double Click {
        n298 = event-data() -> ("PlatMods"=w453:T18, "Tag"=w450:string)  [unwired: 1 in]
        n299 = Unbundle(w453) -> ("Shift"=w452:bool)  [unwired: 4 out]
        n300 = String Subset(string=w450, length (rest)=1 ("length (rest)")) -> (substring=w449:string)  [unwired: 1 in]
        n301 = Not(x=w452) -> (.not. x?=w451:bool)
        n302 = case shown="\"/\"" w449 {
          tunnel: w450 -> [_ w456]
          tunnel: w451 -> [_ w455]
          frame Default {
          }
          frame "/" {
            n303 = call <vilib>:"NT Update Persistence.vi"("Persistence"=w455, "Name"=w456) -> ()  [unwired: 9 in, 1 out]
          }
        }
      }
    }
  }
  n304 = while {
    tunnel: w63 -> [w458]
    i -> [w461]
    stop <- FALSE stop-if-true
    n305 = Wait (ms)(milliseconds to wait=u32 100) -> ()  [unwired: 1 out]
    n306 = case shown="\"Playback\"" "Rec Mode" {
      tunnel: w461 -> [_ _ w476]
      tunnel: [u32 2829099 ("Base Color") u32 11141120 ("Target Color") w465] -> w457
      frame "Stop", Default {
        # "Reset the color, extra updates don't cost much"
      }
      frame "Record" {
      }
      frame "Playback" {
        # "Playback"
        n307 = Quotient & Remainder(x=w476, y=u32 50 ("milliseconds to wait")) -> (x-y*floor(x/y)=w472:u32)  [unwired: 1 out]
        n308 = Divide(x=w472, y=u32 50 ("milliseconds to wait")) -> (x/y=w469:dbl)
        n309 = Multiply(x=6.283185307179586, y=w469) -> (x*y=w474:dbl)
        n310 = Sine(x=w474) -> (sin(x)=w473:dbl)
        n311 = Absolute Value(x=w473) -> (abs(x)=w466:dbl)
        n312 = call "Interpolate RGB Color.vi"("Proportion"=w466, "Target Color"=u32 30976, "Base Color"=u32 2829099) -> ("Result Color"=w465:u32)  [unwired: 8 in]
      }
    }
    n313 = property class="Pane"(reference=w458, "PaneColor"=w457) -> ()  [unwired: 1 in, 2 out]
  }
  n314 = local write "Dashboard Tab"(T2."Drive" ("Dashboard Tab")) -> ()
  n315 = property on="On/Off" class="Bool (strict)"("Visible"=w34) -> ()  [unwired: 2 in, 2 out]
  n316 = property on="Motor" class="Clust (strict)"("Visible"=w34) -> ()  [unwired: 2 in, 2 out]
  n317 = property on="Progress" class="Clust (strict)"("Visible"=w34) -> ()  [unwired: 2 in, 2 out]
  n318 = property on="Test Ring" class="Ring (strict)"("Visible"=w34) -> ()  [unwired: 2 in, 2 out]
  n319 = property on="Rev/Fwd" class="Clust (strict)"("Visible"=w34) -> ()  [unwired: 2 in, 2 out]
  n320 = local write "Command Selection"(u16 0 ("milliseconds to wait")) -> ()
  n321 = while {
    tunnel: u16 1741 ("timeout ms (25000)") -> [w478]
    stop <- FALSE stop-if-true
    n322 = TCP Create Listener(10:w478) -> (0:w477:errorcluster, 3:w479:refnum<k5>)  [unwired: 4 in, 1 out]
    n323 = case shown="No Error" w477 {
      selector: w477 -> [w481 _]
      tunnel: w479 -> [w482 _]
      frame No Error {
        n324 = while {
          tunnel: w482 -> [w485]
          tunnel: w481 -> [w484]
          stop <- FALSE stop-if-true
          n325 = TCP Wait On Listener(8:w484, 11:w485) -> (0:w486:errorcluster, 4:w487:refnum<k5>)  [unwired: 2 in, 3 out]
          n326 = local write "TCP"(w487) -> ()
          n327 = case shown="No Error" w486 {
            frame No Error {
            }
            frame Error {
              n328 = Wait (ms)(milliseconds to wait=u32 1000) -> ()  [unwired: 1 out]
            }
          }
        }
      }
      frame Error {
        n329 = Wait (ms)(milliseconds to wait=u32 1000) -> ()  [unwired: 1 out]
      }
    }
  }
  n330 = local write "Command Params"(string[][] [] ("Command Params")) -> ()
  n331 = global write "WPI_DashboardLogging Global.vi" "Recording"(w57) -> ()
  n332 = local write "Rec Mode"(w57) -> ()
